vi "Stepper L298 Drive_V3.vi"(9 "Start Location Step (-90to90)":i32, 10 "Target Angle (-90to90)":dbl, 11 "stop":bool) -> (1 "Current Motor Step (0to3)":i32)   [LabVIEW 2017]
uses:
  <vilib>/myRIO/Common/Instrument Driver Framework/myRIO v1.0/DIO/typedefs/DIO Channels Enum.ctl
  <vilib>/myRIO/Common/Instrument Driver Framework/myRIO v1.0/DIO/typedefs/DIO Channels List.ctl
  <vilib>/myRIO/Common/Instrument Driver Framework/Utilities/typedefs/Generic FPGA Reference.ctl
  <vilib>/myRIO/Common/Instrument Driver Framework/Utilities/typedefs/myRIO v1.0 Reference.ctl
  <vilib>/myRIO/Common/Instrument Driver Framework/Utilities/typedefs/Hardware Version Enum.ctl
  <vilib>/myRIO/Common/Instrument Driver Framework/Utilities/typedefs/myRIO Generic Hardware Reference.ctl
  <vilib>/myRIO/Instrument Drivers/Onboard IO/DIO/typedefs/DIO Reference.ctl
  <vilib>/myRIO/Instrument Drivers/Onboard IO/DIO/vis/Write.vi
  <vilib>/userdefined/High Color/nirio_resource_hc.ctl
  <vilib>/myRIO/Common/Instrument Driver Framework/myRIO v1.0/DIO/vis/myRIO v1.1 Open DIO.vi
  <vilib>/myRIO/Instrument Drivers/Onboard IO/DIO/vis/myRIO DIO Open.xnode
  <vilib>/myRIO/Common/Instrument Driver Framework/Utilities/vis/Is FPGA Ref Available.vi
  <vilib>/myRIO/Express VI/Onboard IO/DO/DO Express VI.xnode
  <vilib>/myRIO/Express VI/Onboard IO/PWM/PWM Express VI.xnode
  <vilib>/myRIO/Instrument Drivers/Onboard IO/PWM/vis/Set Duty Cycle and Frequency.vi
  <vilib>/myRIO/Instrument Drivers/Onboard IO/PWM/typedefs/PWM Configuration.ctl
  <vilib>/myRIO/Common/Instrument Driver Framework/myRIO v1.0/PWM/typedefs/PWM Channels Enum.ctl
  <vilib>/myRIO/Instrument Drivers/Onboard IO/PWM/typedefs/PWM Reference.ctl
  <vilib>/myRIO/Instrument Drivers/Onboard IO/PWM/vis/myRIO PWM Open.xnode
  <vilib>/myRIO/Common/Instrument Driver Framework/myRIO v1.0/PWM/vis/myRIO v1.1 Open PWM.vi
panel:
  in  "Current Angle (°)":dbl
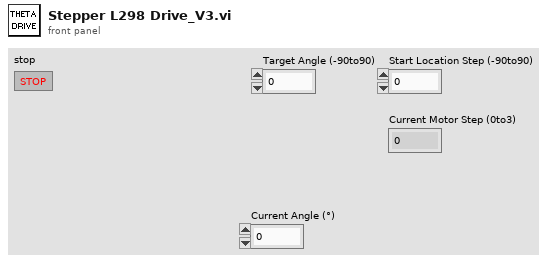
[diagram p1: front panel]
types:
  T1 = typedef "DIO.lvlib/DIO Reference.ctl" = cluster{"myRIO Reference":T2, "DIO Channels List":T6}
  T2 = typedef "myRIO Generic Hardware Reference.ctl" = cluster{"myRIO Model":T3, "myRIO Hardware Reference":T4}
  T3 = typedef "Hardware Version Enum.ctl" = enum16{"Unknown", "myRIO-1900", "myRIO-1950", "roboRIO", "NI ELVIS RIO CM"}
  T4 = typedef "myRIO v1.0 Reference.ctl" = cluster{"Generic FPGA Reference":T5, "Allow multiple opens":bool}
  T5 = typedef "Generic FPGA Reference.ctl" = refnum<k20>
  T6 = typedef "DIO Channels List.ctl" = T7[]
  T7 = typedef "DIO Channels Enum.ctl" = enum16{"Not Connected", "C/DIO0", "C/DIO1", "C/DIO2", "C/DIO3", "C/DIO4", "C/DIO5", "C/DIO6", "C/DIO7", "A/DIO0", "A/DIO1", "A/DIO2", "A/DIO3", "A/DIO4", "A/DIO5", "A/DIO6", "A/DIO7", "A/DIO8", "A/DIO9", "A/DIO10", "A/DIO11", "A/DIO12", "A/DIO13", "A/DIO14", "A/DIO15", "B/DIO0", "B/DIO1", "B/DIO2", "B/DIO3", "B/DIO4", "B/DIO5", "B/DIO6", "B/DIO7", "B/DIO8", "B/DIO9", "B/DIO10", "B/DIO11", "B/DIO12", "B/DIO13", "B/DIO14", "B/DIO15", "LED0", "LED1", "LED2", "LED3", "Button0", "DIO/DIO0", "DIO/DIO1", "DIO/DIO2", "DIO/DIO3", "DIO/DIO4", "DIO/DIO5", "DIO/DIO6", "DIO/DIO7", "DIO/DIO8", "DIO/DIO9", "SPI/CS0", "SPI/CS1", "SPI/CS2", "SPI/CS3", "LED RADIO (Green)", "LED RADIO (Red)", "LED COMM (Green)", "LED COMM (Red)", "LED MODE (Green)", "LED MODE (Red)"}
  T8 = typedef "nirio_resource_hc.ctl" = tag
  T9 = typedef "PWM.lvlib/PWM Reference.ctl" = cluster{"myRIO Reference":T2, "PWM Channels Enum":T10, "PWM Configuration":T11}
  T10 = typedef "PWM Channels Enum.ctl" = enum16{"Not Connected", "C/PWM0", "C/PWM1", "A/PWM0", "A/PWM1", "A/PWM2", "B/PWM0", "B/PWM1", "B/PWM2", "PWM/PWM0", "PWM/PWM1", "PWM/PWM2", "PWM/PWM3", "PWM/PWM4", "PWM/PWM5", "PWM/PWM6", "PWM/PWM7", "PWM/PWM8", "PWM/PWM9"}
  T11 = typedef "PWM.lvlib/PWM Configuration.ctl" = cluster{"Frequency":dbl, "Duty Cycle":dbl}
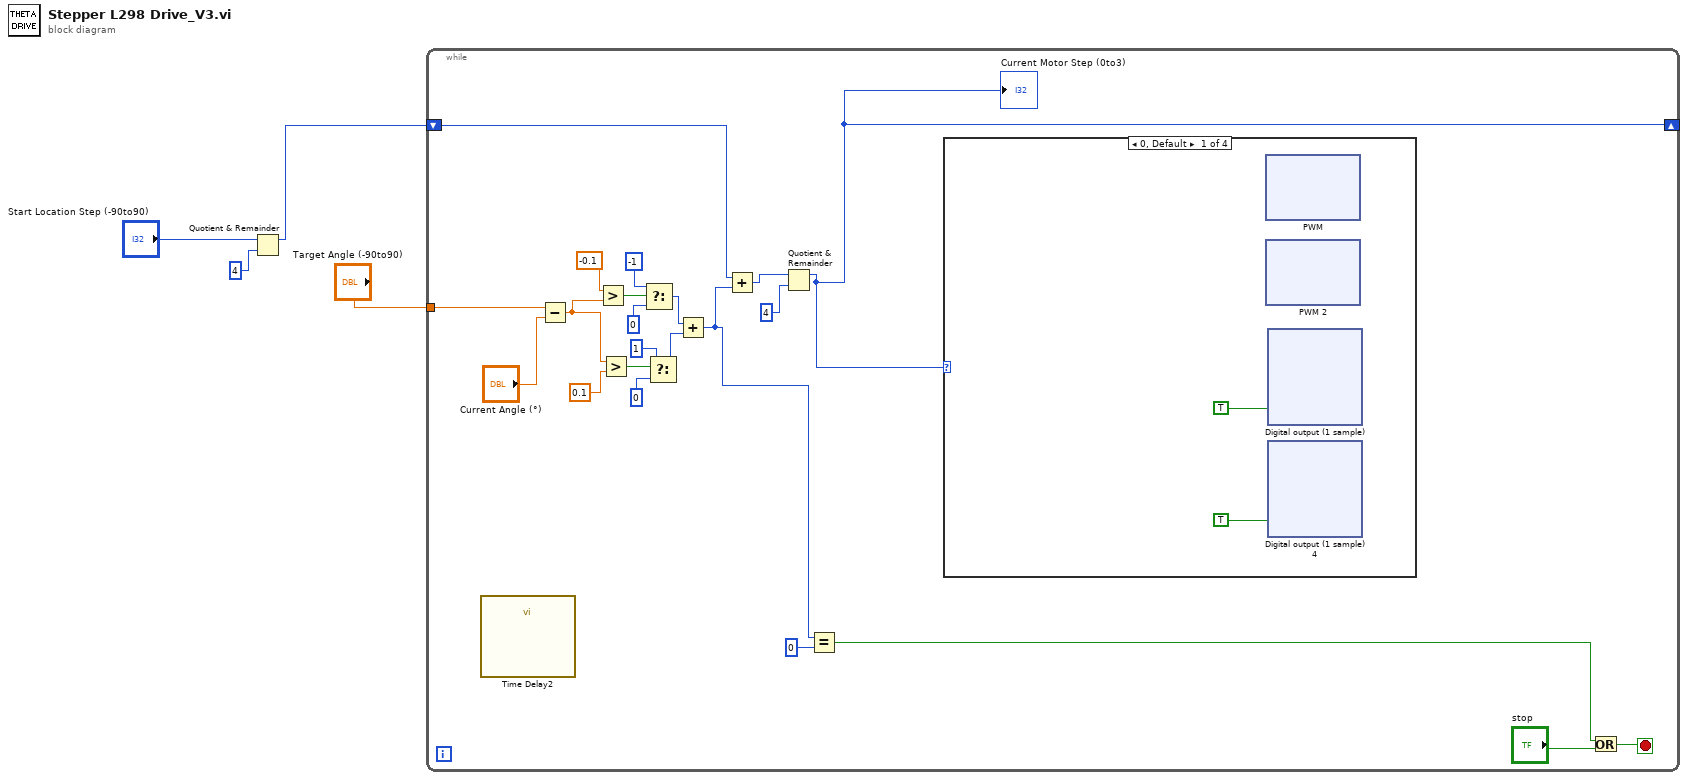
[diagram p0: block diagram]
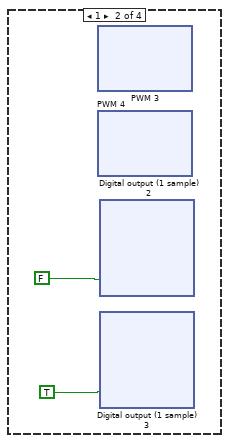
[diagram p2: hidden frame]
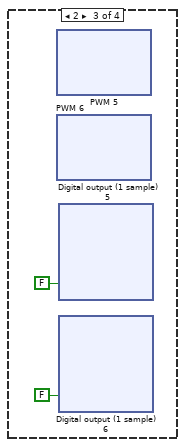
[diagram p3: hidden frame]
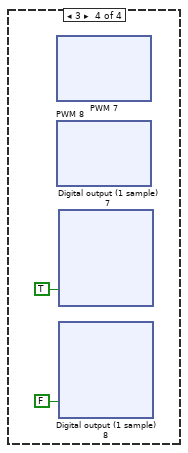
[diagram p4: hidden frame]
diagram:
  n1 = Quotient & Remainder(x="Start Location Step (-90to90)", y=4) -> (x-y*floor(x/y)=w1:i32)  [unwired: 1 out]
  n2 = while {
    tunnel: "Target Angle (-90to90)" -> [w11]
    shift-right: [w12] -> _
    shift-left: w1 -> [w13]
    stop <- w10 stop-if-true
    n3 = call "Time Delay2"() -> ()  [unwired: 11 in, 1 out]
    n4 = Subtract(x=w11, y="Current Angle (°)") -> (x-y=w25:dbl)
    n5 = Greater?(x=-0.1, y=w25) -> (0:w23:bool)
    n6 = Greater?(x=w25, y=0.1) -> (0:w20:bool)
    n7 = Select(t=-1, s=w23, f=0) -> (s? t:f=w17:i32)
    n8 = Select(t=1, s=w20, f=0) -> (s? t:f=w16:i32)
    n9 = Add(x=w17, y=w16) -> (x+y=w6:i32)
    n10 = Add(x=w13, y=w6) -> (x+y=w15:i32)
    n11 = Quotient & Remainder(x=w15, y=4) -> (x-y*floor(x/y)=w12:i32)  [unwired: 1 out]
    "Current Motor Step (0to3)" <- w12
    n12 = Equal?(x=w6, y=0) -> (x = y?=w8:bool)
    n13 = case shown="0, Default" w12 {
      frame 0, Default {
        n14 = xnode "PWM"() -> ()  [unwired: 1 in, 1 out]
        n15 = xnode "PWM 2"() -> ()  [unwired: 1 in, 1 out]
        n16 = xnode "Digital output (1 sample)"("C/DIO5 (DIO5)"=TRUE) -> ()  [unwired: 1 in, 1 out]
        n17 = xnode "Digital output (1 sample) 4"("C/DIO4 (DIO4)"=TRUE) -> ()  [unwired: 1 in, 1 out]
      }
      frame 1 {
        n18 = xnode "PWM 3"() -> ()  [unwired: 1 in, 1 out]
        n19 = xnode "PWM 4"() -> ()  [unwired: 1 in, 1 out]
        n20 = xnode "Digital output (1 sample) 2"("C/DIO5 (DIO5)"=FALSE) -> ()  [unwired: 1 in, 1 out]
        n21 = xnode "Digital output (1 sample) 3"("C/DIO4 (DIO4)"=TRUE) -> ()  [unwired: 1 in, 1 out]
      }
      frame 2 {
        n22 = xnode "PWM 5"() -> ()  [unwired: 1 in, 1 out]
        n23 = xnode "PWM 6"() -> ()  [unwired: 1 in, 1 out]
        n24 = xnode "Digital output (1 sample) 5"("C/DIO5 (DIO5)"=FALSE) -> ()  [unwired: 1 in, 1 out]
        n25 = xnode "Digital output (1 sample) 6"("C/DIO4 (DIO4)"=FALSE) -> ()  [unwired: 1 in, 1 out]
      }
      frame 3 {
        n26 = xnode "PWM 7"() -> ()  [unwired: 1 in, 1 out]
        n27 = xnode "PWM 8"() -> ()  [unwired: 1 in, 1 out]
        n28 = xnode "Digital output (1 sample) 7"("C/DIO5 (DIO5)"=TRUE) -> ()  [unwired: 1 in, 1 out]
        n29 = xnode "Digital output (1 sample) 8"("C/DIO4 (DIO4)"=FALSE) -> ()  [unwired: 1 in, 1 out]
      }
    }
    n30 = Or(x=w8, y="stop") -> (x .or. y?=w10:bool)
  }
